vi "RX_RY_write.vi"(1 "Barcode":string, 2 "CAN_MSGs_Write":T1={"Scaling Factor"=1, "Physical value"=0.0, "CAN_Frames"={"CAN_ID"=0, "MSGTYPE"=128, "Payload"=[], "Length"=0}, "Offset value"=0.0, "Framing datas"=[], "CAN_Frame Enable"=FALSE, "Add Signal"=FALSE, "Delete Signal"=FALSE, "Signal Values"=[], "Time(ms)"=0.0, "Repetition"=FALSE, "Delay"=FALSE, "Delay time"=0.0} {"CAN_Frames"."Payload" format="%.0x"; "CAN_Frames"."MSGTYPE" items=["STATUS"=128, "EXTENDED"=2, "RTR"=1, "DATA MSG"=0]; "CAN_Frames"."CAN_ID" format="%.0x"}) -> (0 "CAN_msgs":T1={"Scaling Factor"=1, "Physical value"=0.0, "CAN_Frames"={"CAN_ID"=0, "MSGTYPE"=128, "Payload"=[], "Length"=0}, "Offset value"=0.0, "Framing datas"=[], "CAN_Frame Enable"=FALSE, "Add Signal"=FALSE, "Delete Signal"=FALSE, "Signal Values"=[], "Time(ms)"=0.0, "Repetition"=FALSE, "Delay"=FALSE, "Delay time"=0.0} {"CAN_Frames"."Payload" format="%.0x"; "CAN_Frames"."MSGTYPE" items=["STATUS"=128, "EXTENDED"=2, "RTR"=1, "DATA MSG"=0]; "CAN_Frames"."CAN_ID" format="%.0x"})   [LabVIEW 2024]
uses:
  PCANusb_DTU/support/CAN_Frames_ctrl.ctl
  PCANusb_DTU/PCANusb_DTU.lvlib
  PCANusb_DTU/support/Framing datas.ctl
  PCANusb_DTU/support/CAN_MSGs.ctl
panel:
  out "number":u8
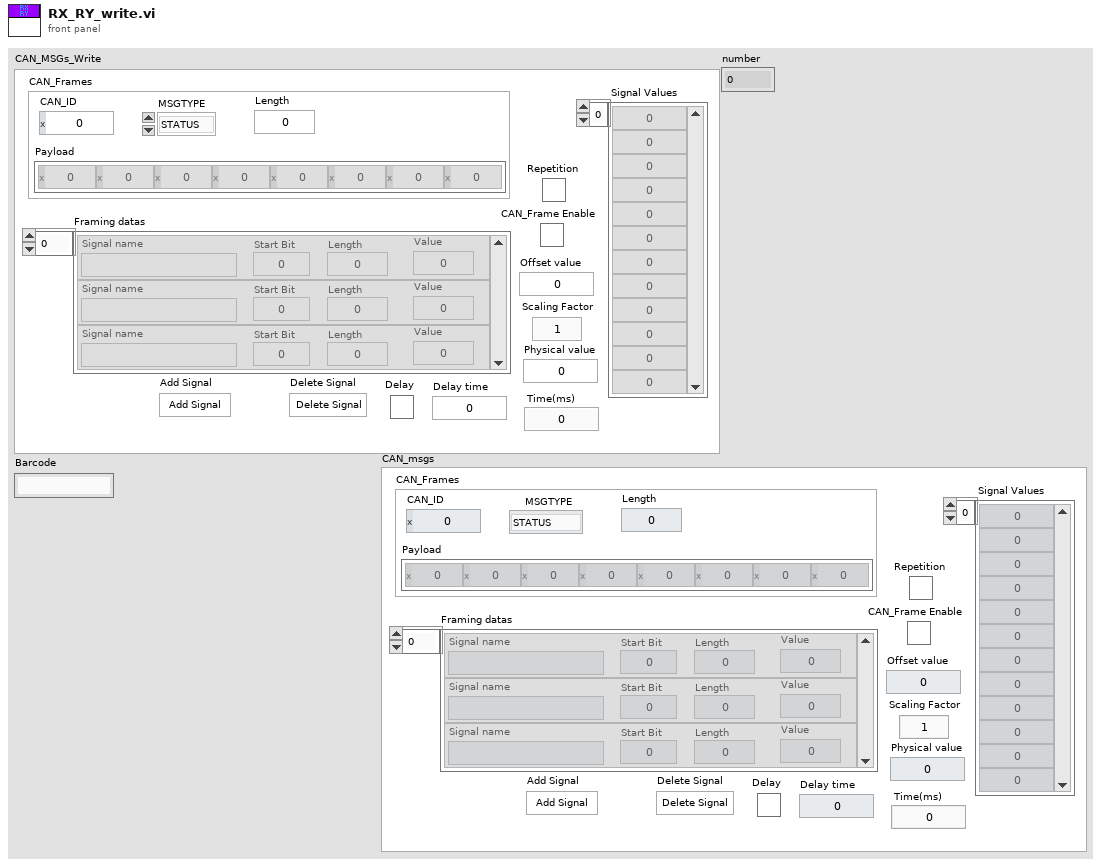
[diagram p1: front panel]
types:
  T1 = typedef "PCANusb_DTU.lvlib/CAN_MSGs.ctl" = cluster{"Scaling Factor":u16, "Physical value":dbl, "CAN_Frames":T2, "Offset value":dbl, "Framing datas":T3[], "CAN_Frame Enable":bool, "Add Signal":bool, "Delete Signal":bool, "Signal Values":dbl[], "Time(ms)":dbl, "Repetition":bool, "Delay":bool, "Delay time":dbl}
  T2 = typedef "PCANusb_DTU.lvlib/CAN_Frames_ctrl.ctl" = cluster{"CAN_ID":u32, "MSGTYPE":u8, "Payload":u8[], "Length":u8}
  T3 = typedef "PCANusb_DTU.lvlib/Framing datas.ctl" = cluster{"Signal name":string, "Start Bit":u8, "Length":u8, "Value":u16}
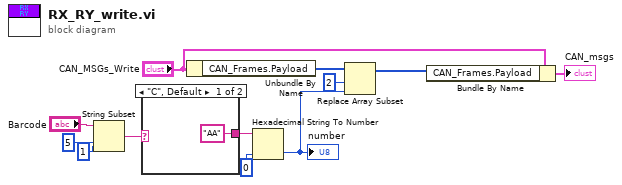
[diagram p0: block diagram]
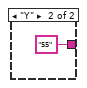
[diagram p2: hidden frame]
diagram:
  n1 = String Subset(string="Barcode", offset (0)=5, length (rest)=1 ("length (rest)")) -> (substring=w9:string)
  n2 = case shown="\"C\", Default" w9 {
    tunnel: ["AA" "55"] -> w8
    frame "C", Default {
    }
    frame "Y" {
    }
  }
  n3 = Unbundle By Name("CAN_MSGs_Write") -> ("CAN_Frames.Payload"=w6:u8[])
  n4 = Hexadecimal String To Number(string=w8, default (0uL)=u8 0) -> (number=w4:u8)  [unwired: 1 in, 1 out]
  "number" <- w4
  n5 = Replace Array Subset(array=w6, new element=w4, index=2) -> (w2:u8[])
  n6 = Bundle By Name(cluster="CAN_MSGs_Write", "CAN_Frames.Payload"=w2) -> (→"CAN_msgs":T1)
